vi "Lake Shore Cryotronics 331 Application Curve.vi"(1 "Curve (21)":dbl=21.0 min=21.0 max=41.0 step=1.0, 2 "Write Curve Header (F: Don't Write Header)":bool, 3 "Curve Serial Number (\"\")":string, 4 "Limit Value (0.000)":dbl min=0.0 max=1500.0 step=0.001 format="%.3f", 6 "Write Curve\nPoint (F: Don't Write Point)":bool, 7 "Curve Name (\"\")":string, 8 "Index (1)":dbl=1.0 min=1.0 max=200.0 step=1.0, 9 "Curve Data Format (0: mV/K)":u16(ring) items=["mV/K", "V/K", "Ohms/K", "Log Ohms/K"], 10 "Temperature \nValue (0.0000)":dbl min=-9999.0 max=9999.0 step=1e-05 format="%.4f", 11 "Temp Coefficient (0: Negative)":u16(ring) items=["Negative", "Positive"], 12 "Units Value (0.00000)":dbl min=-9999.0 max=9999.0 step=1e-05 format="%.5f") -> ()   [LabVIEW 2010]
doc: "This vi was designed to demonstrate typical usage of sub vi's containing the 331 curve functions.\n\nThis vi performs 2 curve functions, write curve header, and write curve point. A typical way to use this vi would be to first write a curve header, then write multiple curve points until all points are written."
uses:
  <instrlib>/Lake Shore Cryotronics 331/Lake Shore Cryotronics 331.lvlib
panel:
  in  "VISA resource name":refnum<visa-resource-name>
  # "(c) 2007-2009 Lake Shore Cryotronics Inc.  ALL RIGHTS RESERVED."
  # "Write Header\nDon't Write Header"
  # "Write Point\nDon't Write Point"
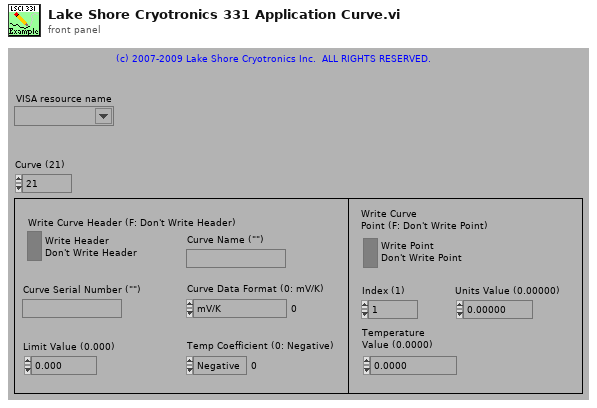
[diagram p1: front panel]
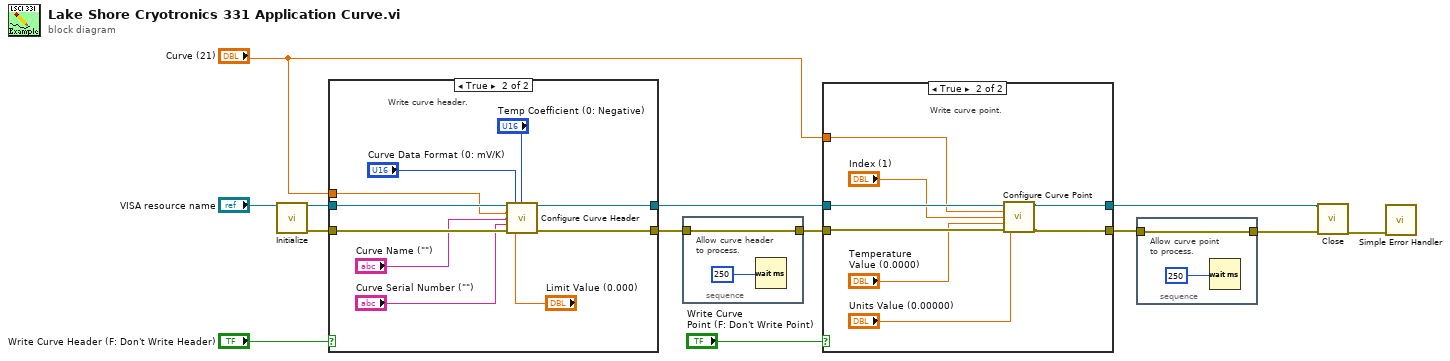
[diagram p0: block diagram]
diagram:
  n1 = call <instrlib>:"Initialize.vi"("VISA resource name"="VISA resource name") -> ("VISA resource name out"=w7:refnum<visa-resource-name>, "error out"=w6:errorcluster)  [unwired: 13 in]
  n2 = case shown="True" "Write Curve Header (F: Don't Write Header)" {
    tunnel: w7 -> [w15 w22]
    tunnel: w6 -> [w14 w23]
    tunnel: [w15 w25] -> w12
    tunnel: [w14 w24] -> w10
    tunnel: "Curve (21)" -> [_ w19]
    frame False {
      # "Don't write curve header."
    }
    frame True {
      # "Write curve header."
      n3 = call <instrlib>:"Configure Curve Header.vi"("VISA resource name"=w22, "Curve Data Format (0: mV/K)"="Curve Data Format (0: mV/K)", "Temp Coefficient (0: Negative)"="Temp Coefficient (0: Negative)", "Curve (21)"=w19, "Curve Name (\"\")"="Curve Name (\"\")", "Curve Serial Number (\"\")"="Curve Serial Number (\"\")", "error in (no error)"=w23, "Limit Value (0.000)"="Limit Value (0.000)") -> ("VISA resource name out"=w25:refnum<visa-resource-name>, "error out"=w24:errorcluster)  [unwired: 6 in]
    }
  }
  n4 = stacked-sequence {
    tunnel: w10 -> [w26]
    tunnel: [w26] -> w9
    frame #0 {
      # "Allow curve header\nto process."
      n5 = Wait (ms)(milliseconds to wait=u32 250) -> ()  [unwired: 1 out]
    }
  }
  n6 = case shown="True" "Write Curve\nPoint (F: Don't Write Point)" {
    tunnel: w12 -> [w29 w37]
    tunnel: w9 -> [w28 w34]
    tunnel: "Curve (21)" -> [_ w30]
    tunnel: [w29 w36] -> w3
    tunnel: [w28 w35] -> w4
    frame False {
      # "Don't Write curve point."
    }
    frame True {
      # "Write curve point."
      n7 = call <instrlib>:"Configure Curve Point.vi"("VISA resource name"=w37, "Curve (21)"=w30, "Index (1)"="Index (1)", "Temperature \nValue (0.0000)"="Temperature \nValue (0.0000)", "error in (no error)"=w34, "Units Value (0.00000)"="Units Value (0.00000)") -> ("VISA resource name out"=w36:refnum<visa-resource-name>, "error out"=w35:errorcluster)  [unwired: 8 in]
    }
  }
  n8 = stacked-sequence {
    tunnel: w4 -> [w38]
    tunnel: [w38] -> w2
    frame #0 {
      # "Allow curve point\nto process."
      n9 = Wait (ms)(milliseconds to wait=u32 250) -> ()  [unwired: 1 out]
    }
  }
  n10 = call <instrlib>:"Close.vi"("VISA resource name"=w3, "error in (no error)"=w2) -> ("error out"=w1:errorcluster)  [unwired: 13 in]
  n11 = call <vilib>:"Simple Error Handler.vi"("error in (no error)"=w1) -> ()  [unwired: 4 in, 5 out]
